vi "Build Channel Configuration.vi"(8 "error in (no error)":errorcluster, 11 "PicoScope 3000a in":refnum<class "PicoScope 3000a.lvclass">) -> (0 "error out":errorcluster, 1 "Channel Numbers":u32[](array[numeric]), 3 "PicoScope 3000a out":refnum<class "PicoScope 3000a.lvclass">)   [LabVIEW 2018, in "PicoScope 3000a.lvlib" / "PicoScope 3000a.lvclass"]
uses:
  PicoScope 3000a.lvclass
  PicoScope 3000a.lvclass/PicoScope 3000a.ctl
  LWS SLA-070/Distro/Projects/12170 Luminar LWS Base/Source/PPLs/Configuration.lvlibp/Configuration.lvclass
  LWS SLA-070/Distro/Projects/12170 Luminar LWS Base/Source/PPLs/Oscilloscope.lvlibp/Oscilloscope.lvclass
  C:/Projects/LWS SLA-070/Distro/Projects/12170 Luminar LWS Base/Source/PPLs/Oscilloscope.lvlibp/Oscilloscope.lvclass
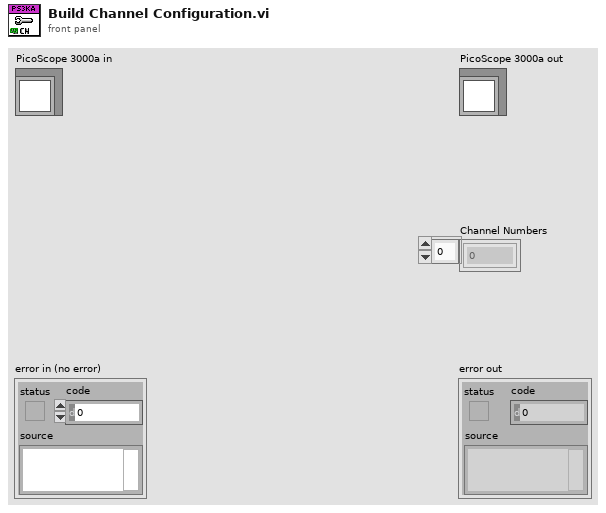
[diagram p1: front panel]
types:
  T1 = cluster{"Enabled":bool, "Coupling":u32, "Range":u32, "Analogue Offset":sgl}
  T2 = cluster{"Channel":enum16{"CH. A", "CH. B", "CH. C", "CH. D"}, "Range":u32}
  T3 = cluster{"Channel":enum16{"CH. A", "CH. B", "CH. C", "CH. D"}, "Range":u32}[]
  T4 = cluster{"Driver Version":string, "USB Version":string, "Hardware":string, "Variant":string, "Batch and Serial":string, "Cal Date":string, "Kernel Version":string, "Digital HW Version":string, "Analogue HW Version":string, "MSO":bool, "Number of channels":i16}
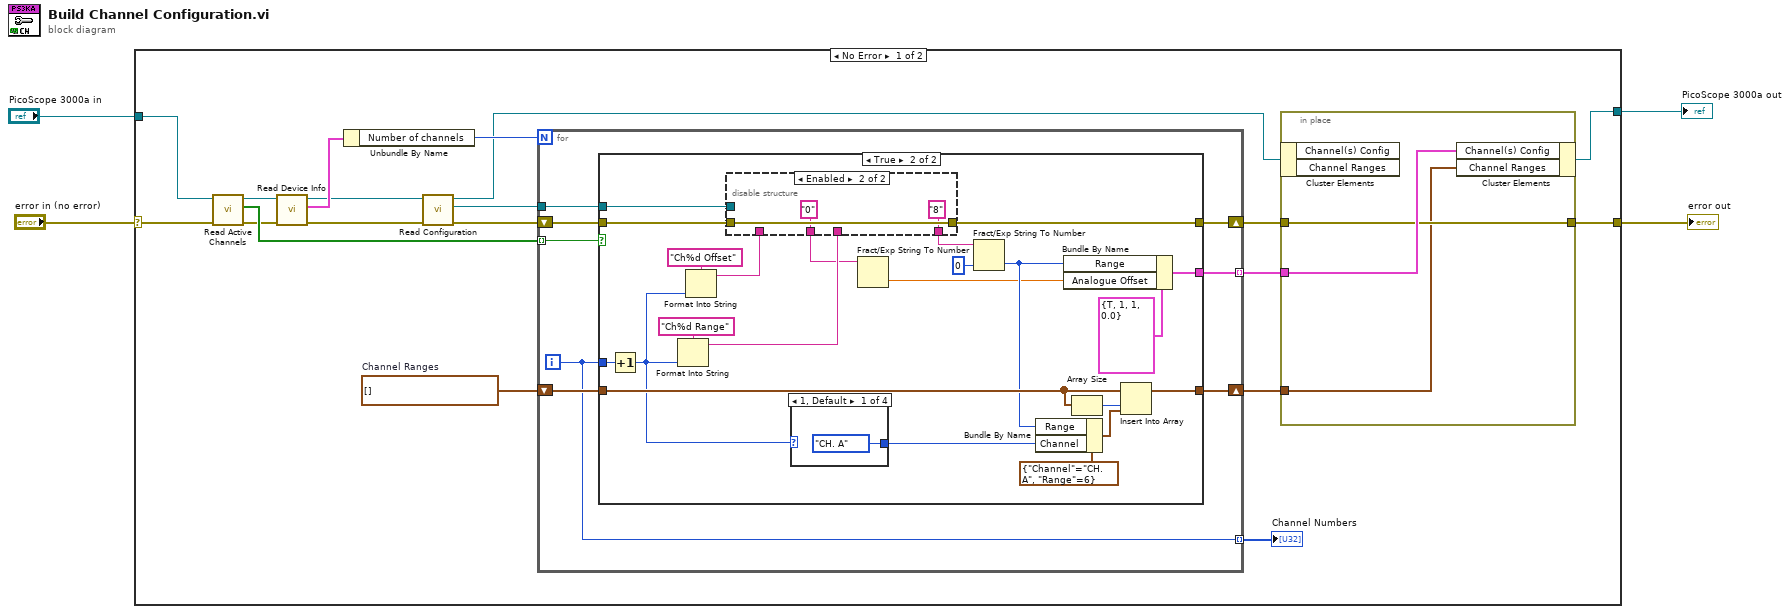
[diagram p0: block diagram]
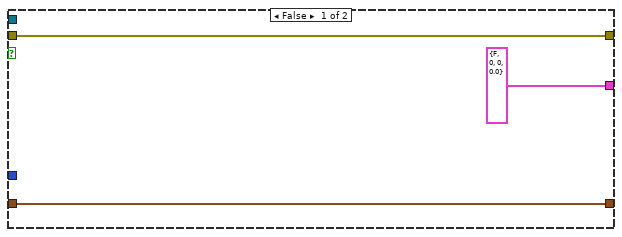
[diagram p2: hidden frame]
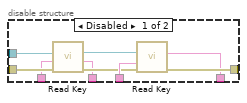
[diagram p3: hidden frame]
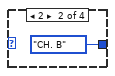
[diagram p4: hidden frame]
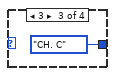
[diagram p5: hidden frame]
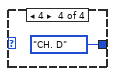
[diagram p6: hidden frame]
diagram:
  n1 = case shown="No Error" "error in (no error)" {
    selector: "error in (no error)" -> [w23 w77]
    tunnel: [w16 w77] -> w3
    tunnel: [w5 w76] -> w1
    tunnel: "PicoScope 3000a in" -> [w22 w76]
    frame No Error {
      w18 = T3 []  # Channel Ranges
      n2 = call "Read Active Channels.vi"("error in (no error)"=w23, "PicoScope 3000a in"=w22) -> ("error out"=w14:errorcluster, "Active Channels"=w21:bool[], "PicoScope 3000a out"=w15:refnum<class "PicoScope 3000a.lvclass">)  [unwired: 7 in]
      n3 = call "Read Device Info.vi"("error in (no error)"=w14, "PicoScope 3000a in"=w15) -> ("error out"=w10:errorcluster, "Device Info"=w13:T4, "PicoScope 3000a out"=w11:refnum<class "PicoScope 3000a.lvclass">)  [unwired: 7 in]
      n4 = Unbundle By Name(w13) -> ("Number of channels"=w12:i16)
      n5 = call "Read Configuration.vi"("error in (no error)"=w10, "Oscilloscope in"=w11) -> ("error out"=w20:errorcluster, "Configuration"=w19:refnum<class "Configuration.lvclass">, "Oscilloscope out"=w6:refnum<class "PicoScope 3000a.lvclass">)  [unwired: 7 in]
      n6 = for {
        N: w12 -> [_]
        tunnel: w21 -> [w34] mode=indexing
        tunnel: w19 -> [w32]
        shift-right: [w31] -> w7
        shift-left: w20 -> [w33]
        tunnel: [w30] -> w8 mode=indexing
        shift-right: [w28] -> w17
        shift-left: w18 -> [w29]
        tunnel: [w27] -> w9 mode=indexing
        i -> [w27]
        n7 = case shown="True" w34 {
          tunnel: w33 -> [w37 w58]
          tunnel: w32 -> [_ w59]
          tunnel: w27 -> [_ w46]
          tunnel: [w37 w54] -> w31
          tunnel: [T1 {"Enabled"=FALSE, "Coupling"=0, "Range"=0, "Analogue Offset"=0.0} ("Channel A Settings") w53] -> w30
          tunnel: w29 -> [w35 w51]
          tunnel: [w35 w50] -> w28
          frame False {
          }
          frame True {
            n8 = Increment(x=w46) -> (x+1=w44:i32)
            n9 = Format Into String(format string="Ch%d Range", w44) -> (resulting string=w43:string)  [unwired: 2 in, 1 out]
            n10 = Format Into String(format string="Ch%d Offset", w44) -> (resulting string=w56:string)  [unwired: 2 in, 1 out]
            n11 = disable-structure shown="Enabled" {
              disable-tunnel: w59 -> [w68 _]
              disable-tunnel: w58 -> [w67 w71]
              disable-tunnel: w56 -> [w66 _]
              disable-tunnel: [w65 w71] -> w54
              disable-tunnel: w43 -> [w64 _]
              disable-tunnel: [w63 "8" ("Value")] -> w42
              disable-tunnel: [w60 "0" ("Value")] -> w39
              frame Disabled {
                n12 = call "Read Key.vi"("Key:"=w66, "error in"=w67, "Configuration in"=w68) -> ("error out"=w61:errorcluster, "Value"=w60:string, "Configuration out"=w62:refnum<class "Configuration.lvclass">)  [unwired: 6 in]
                n13 = call "Read Key.vi"("Key:"=w64, "error in"=w61, "Configuration in"=w62) -> ("error out"=w65:errorcluster, "Value"=w63:string)  [unwired: 6 in, 1 out]
              }
              frame Enabled {
              }
            }
            n14 = case shown="1, Default" w44 {
              tunnel: [enum16{"CH. A", "CH. B", "CH. C", "CH. D"}."CH. A" ("Channel") enum16{"CH. A", "CH. B", "CH. C", "CH. D"}."CH. B" ("Channel") enum16{"CH. A", "CH. B", "CH. C", "CH. D"}."CH. C" ("Channel") enum16{"CH. A", "CH. B", "CH. C", "CH. D"}."CH. D" ("Channel")] -> w48
              frame 1, Default {
              }
              frame 2 {
              }
              frame 3 {
              }
              frame 4 {
              }
            }
            n15 = Fract/Exp String To Number(string=w39) -> (number=w38:dbl)  [unwired: 3 in, 1 out]
            n16 = Fract/Exp String To Number(string=w42, default (0 dbl)=u32 0 ("default (0 DBL)")) -> (number=w40:u32)  [unwired: 2 in, 1 out]
            n17 = Bundle By Name(cluster=T2 {"Channel"=enum."CH. A", "Range"=6} ("Channel Range"), "Range"=w40, "Channel"=w48) -> (w47:T2)
            n18 = Bundle By Name(cluster=T1 {"Enabled"=TRUE, "Coupling"=1, "Range"=1, "Analogue Offset"=0.0} ("Channel A Settings"), "Range"=w40, "Analogue Offset"=w38) -> (w53:T1)
            n19 = Array Size(array=w51) -> (size(s)=w52:i32)
            n20 = Insert Into Array(array=w51, index=w52, new element=w47) -> (w50:T3)
          }
        }
      }
      "Channel Numbers" <- w9
      n21 = in-place {
        in-place-border: w17 -> [w24]
        in-place-border: [w25] -> w16
        in-place-border: w8 -> [w26]
        in-place-border: w7 -> [w25]
        n22 = in-place-cluster #1(w6) -> ()  [unwired: 2 out]
        n23 = in-place-cluster #1("Channel(s) Config"=w26, "Channel Ranges"=w24) -> (w5:refnum<class "PicoScope 3000a.lvclass">)
      }
    }
    frame Error {
    }
  }
  "error out" <- w3
  "PicoScope 3000a out" <- w1
